vi "ep_Reshape Data.vi"(0 "sampling rate in":dbl[](array[numeric]), 5 "appended signal":dbl[][](array[numeric]), 7 "timestamp":timestamp, 9 "system info in":refnum<class "EP System Info.lvclass">, 11 "error in (no error)":errorcluster, 12 "cycles per block":u16, 13 "input cycles":i32, 14 "input size":i32) -> (4 "sampling rate out":dbl[](array[numeric]), 6 "remained signal":dbl[][](array[numeric]), 8 "output data blocks":T1[](array[typedef]), 10 "system info out":refnum<class "EP System Info.lvclass">, 15 "error out":errorcluster)   [LabVIEW 2013, in "NI_EP_Power Quality.lvlib"]
uses:
  <vilib>/addons/Electrical Power/PQ/Common/Classes/System Info/EP System Info.lvclass
  <vilib>/addons/Electrical Power/PQ/Resampling/Desktop/subVIs/ep_Resampled Data.ctl
  <vilib>/Analysis/baseanly.llb/Mean (DBL).vi
  <vilib>/addons/Electrical Power/PQ/NI_EP_Power Quality.lvlib
  <vilib>/Analysis/NI_AALBase.lvlib
  <vilib>/addons/Electrical Power/PQ/Resampling/NI_EP_Resample_Host.lvlib
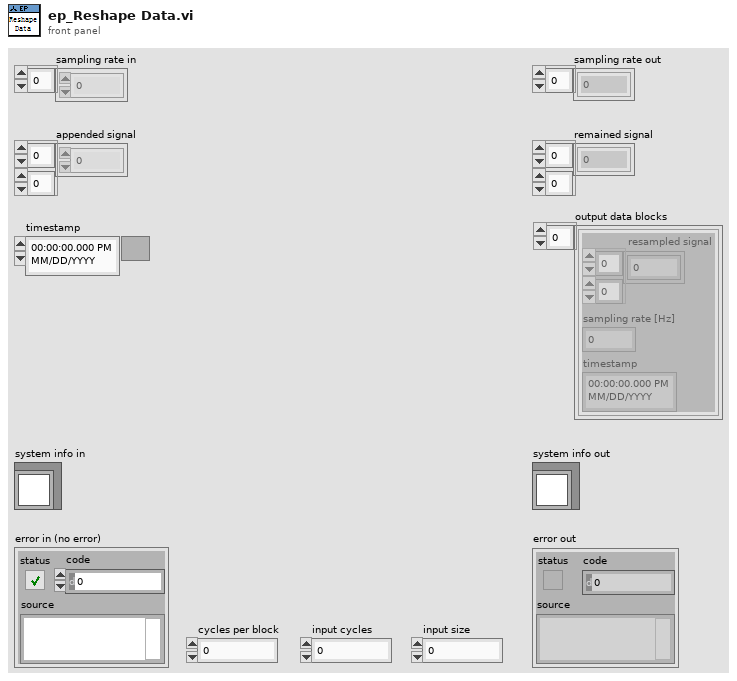
[diagram p1: front panel]
types:
  T1 = typedef "NI_EP_Resample_Host.lvlib/ep_Resampled Data.ctl" = cluster{"resampled signal":dbl[][], "sampling rate [Hz]":dbl, "timestamp":timestamp}
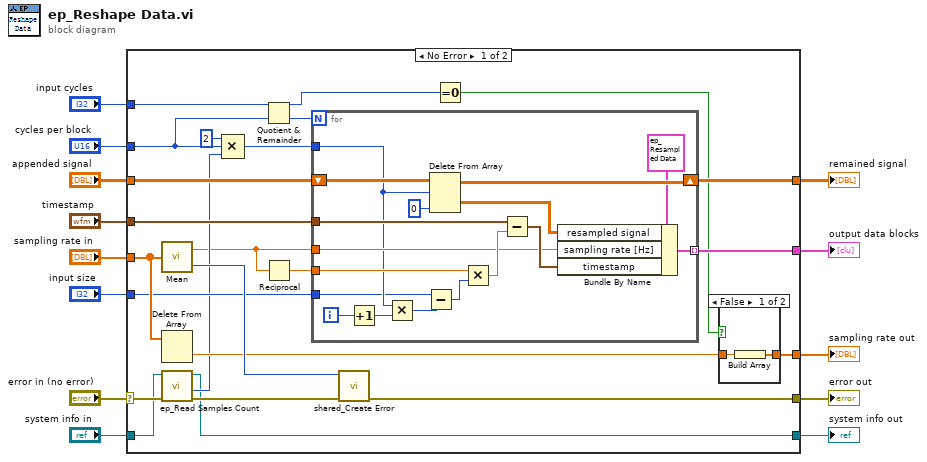
[diagram p0: block diagram]
diagram:
  n1 = case shown="No Error" "error in (no error)" {
    selector: "error in (no error)" -> [w21 w57]
    tunnel: "system info in" -> [w16 w58]
    tunnel: [w15 w58] -> w12
    tunnel: "sampling rate in" -> [w36 _]
    tunnel: "timestamp" -> [w35 _]
    tunnel: [w34 w57] -> w9
    tunnel: [w32 _] -> w8
    tunnel: "appended signal" -> [w30 _]
    tunnel: "input size" -> [w29 _]
    tunnel: "cycles per block" -> [w19 _]
    tunnel: "input cycles" -> [w27 _]
    tunnel: [w26 _] -> w3
    tunnel: [w24 _] -> w2
    frame No Error {
      n2 = call-poly <vilib>:"Mean.vi"("X"=w36) -> ("mean"=w14:dbl, "error"=w33:i32)
      n3 = Delete From Array(array=w36) -> (deleted portion=w25:dbl)  [unwired: 2 in, 1 out]
      n4 = call <vilib>:"ep_Read Samples Count.vi"("error in (no error)"=w21, "system info in"=w16) -> ("error out"=w20:errorcluster, "half-cycle (samples)"=w18:i32, "system info out"=w15:refnum<class "EP System Info.lvclass">)  [unwired: 5 in, 2 out]
      n5 = Compound Arithmetic op=MULTIPLY(2 ("value"), w19, w18) -> (w37:i32)
      n6 = Quotient & Remainder(x=w27, y=w19) -> (x-y*floor(x/y)=w23:i32, floor(x/y)=w28:i32)
      n7 = Reciprocal(x=w14) -> (1/x=w31:dbl)
      n8 = for {
        N: w28 -> [_]
        shift-right: [w56] -> w26
        shift-left: w30 -> [w55]
        tunnel: w37 -> [w46]
        tunnel: w14 -> [w50]
        tunnel: w35 -> [w54]
        tunnel: [w40] -> w32 mode=indexing
        tunnel: w31 -> [w49]
        tunnel: w29 -> [w44]
        i -> [w48]
        n9 = Increment(x=w48) -> (x+1=w47:i32)
        n10 = Multiply(x=w46, y=w47) -> (x*y=w45:i32)
        n11 = Subtract(x=w44, y=w45) -> (x-y=w43:i32)
        n12 = Delete From Array(array=w55, length=w46, index (col)=0 ("disabled index (col)")) -> (deleted portion=w41:dbl[][], array with subset deleted=w56:dbl[][])  [unwired: 1 in]
        n13 = Multiply(x=w49, y=w43) -> (x*y=w52:dbl)
        n14 = Subtract(x=w54, y=w52) -> (x-y=w51:timestamp)
        n15 = Bundle By Name(cluster=T1 {"resampled signal"=[], "sampling rate [Hz]"=0.0, "timestamp"=timestamp(0 s since 1904-01-01)} ("resampled data"), "resampled signal"=w41, "sampling rate [Hz]"=w50, "timestamp"=w51) -> (w40:T1)
      }
      n16 = call <vilib>:"shared_Create Error.vi"("error in (no error)"=w20, "error code (0)"=w33) -> ("error out"=w34:errorcluster)  [unwired: 9 in]
      n17 = Equal To 0?(x=w23) -> (x = 0?=w22:bool)
      n18 = case shown="False" w22 {
        tunnel: w25 -> [w39 _]
        tunnel: [w38 _] -> w24
        frame False {
          n19 = Build Array(w39) -> (w38:dbl[])
        }
        frame True {
        }
      }
    }
    frame Error {
    }
  }
  "system info out" <- w12
  "output data blocks" <- w8
  "sampling rate out" <- w2
  "remained signal" <- w3
  "error out" <- w9
